vi "Image Source.vi"(7 "HTML Destination":path=path "", 8 "Error In":errorcluster, 11 "Spaced File Stem":string) -> (0 "Error Out":errorcluster, 2 "VI Image File":path, 3 "VI Image Src":string)   [LabVIEW 2018, in "Scripts.lvlib"]
uses:
  Scripts.lvlib
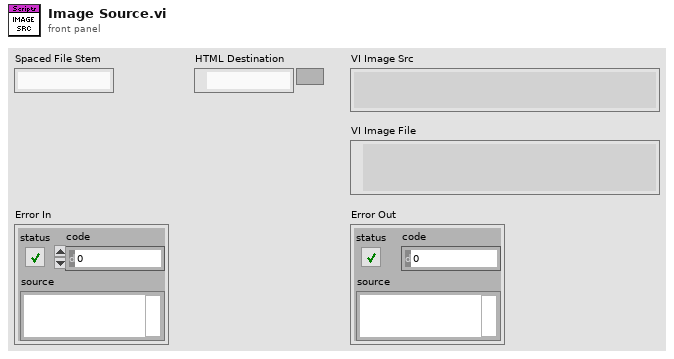
[diagram p1: front panel]
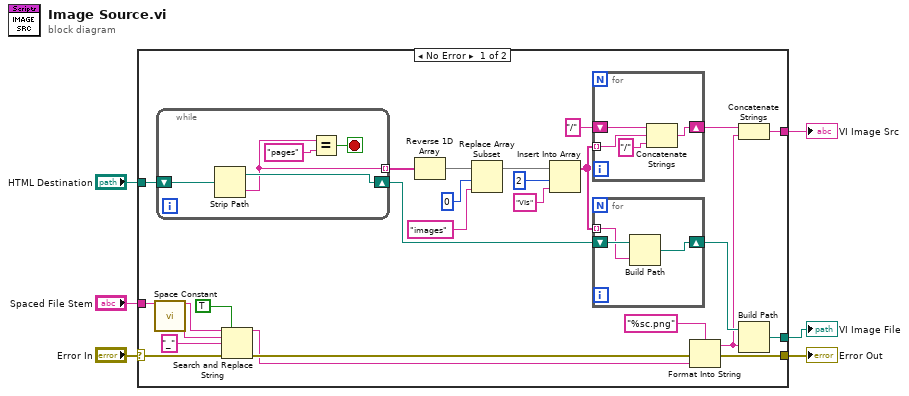
[diagram p0: block diagram]
diagram:
  n1 = case shown="No Error" "Error In" {
    selector: "Error In" -> [w25 w44]
    tunnel: "Spaced File Stem" -> [w31 _]
    tunnel: [w27 w44] -> w5
    tunnel: [w15 _] -> w4
    tunnel: "HTML Destination" -> [w20 _]
    tunnel: [w14 _] -> w1
    frame No Error {
      n2 = call <vilib>:"Space Constant.vi"() -> ("String"=w29:string)
      n3 = while {
        shift-right: [w36] -> w19
        shift-left: w20 -> [w39]
        tunnel: [w35] -> w21 mode=indexing
        stop <- w37 stop-if-true
        n4 = Strip Path(path=w39) -> (stripped path=w36:path, name=w35:string)
        n5 = Equal?(x=w35, y="pages") -> (x = y?=w37:bool)
      }
      n6 = Search and Replace String(replace all?=TRUE ("replace all? (F)"), input string=w31, search string=w29, replace string="_" ("replace string (\"\")"), error in=w25) -> (result string=w22:string, error out=w30:errorcluster)  [unwired: 3 in, 2 out]
      n7 = Reverse 1D Array(array=w21) -> (reversed array=w13:string[])
      n8 = Replace Array Subset(array=w13, new element="images" ("new element/subarray"), index=0) -> (w10:string[])
      n9 = Insert Into Array(array=w10, index=2, new element="VIs" ("new element/subarray")) -> (w7:string[])
      n10 = for {
        shift-right: [w42] -> w17
        shift-left: "/" -> [w43]
        tunnel: w7 -> [w40] mode=indexing
        n11 = Concatenate Strings(w43, w40, "/" ("string")) -> (w42:string)
      }
      n12 = for {
        shift-right: [w33] -> w18
        shift-left: w19 -> [w34]
        tunnel: w7 -> [w32] mode=indexing
        n13 = Build Path(base path=w34, name or relative path=w32) -> (appended path=w33:path)
      }
      n14 = Format Into String(format string="%sc.png", error in=w30, w22) -> (resulting string=w16:string, error out=w27:errorcluster)  [unwired: 1 in]
      n15 = Concatenate Strings(w17, w16) -> (w15:string)
      n16 = Build Path(base path=w18, name or relative path=w16) -> (appended path=w14:path)
    }
    frame Error {
    }
  }
  "Error Out" <- w5
  "VI Image Src" <- w4
  "VI Image File" <- w1
